vi "Filter ConfigurationView.vi"(9 "Stop Event":refnum<user-event>, 10 "Current Filter Settings":T1={"Level Filter"={"Warning"=FALSE, "Debug"=FALSE, "Info"=FALSE, "Error"=FALSE, "Critical"=FALSE}, "Source Filter"={"Source"="", "Exclude Match?"=TRUE, "Exact Match?"=TRUE}, "Keyword Filter"={"Keywords"=[], "Exclude Match?"=TRUE}}, 11 "ViewQueue":refnum<queue>) -> ()   [LabVIEW 2019, in "ConsoleView.lvlib" / "ConsoleView.lvclass"]
uses:
  <vilib>/gpm_packages/@cs/event-logger/Source/ConsoleView/View/ConsoleView.lvclass
  <vilib>/gpm_packages/@cs/event-logger/Source/Composed Log/Types/MessageCluster.ctl
  <vilib>/gpm_packages/@cs/event-logger/Source/ConsoleView/View/TypeDef/FilterConfig.ctl
  <vilib>/gpm_packages/@cs/event-logger/Source/Composed Log/Composed Log.lvlib
panel:
  in  "Cancel":bool
  in  "Apply Changes":bool
  in  "Exclude Keyword Matches?":bool caption="Exclude Matches?"
  in  "Exclude Source Matches?":bool caption="Exclude Matches?"
  in  "Exact Match?":bool
  in  "Keywords":string
  in  "Event Source":string
  in  "Critical":bool
  in  "Error":bool
  in  "Warning":bool
  in  "Info":bool
  in  "Debug":bool
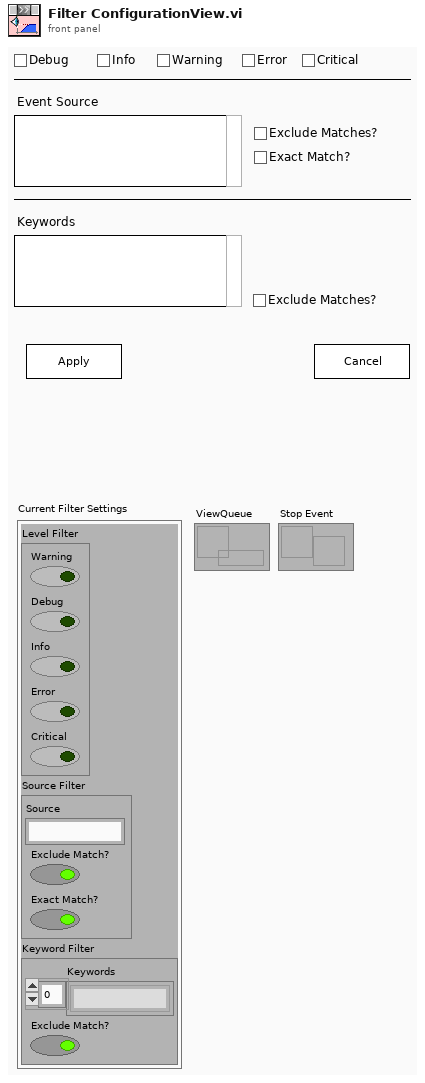
[diagram p1: front panel]
types:
  T1 = typedef "ConsoleView.lvlib/ConsoleView.lvclass/FilterConfig.ctl" = cluster{"Level Filter":cluster{"Warning":bool, "Debug":bool, "Info":bool, "Error":bool, "Critical":bool}, "Source Filter":cluster{"Source":string, "Exclude Match?":bool, "Exact Match?":bool}, "Keyword Filter":cluster{"Keywords":string[], "Exclude Match?":bool}}
  T2 = enum32{"Invalid", "Standard", "Closed", "Hidden", "Minimized", "Maximized"}
  T3 = typedef "Composed Log.lvlib/MessageCluster.ctl" = cluster{"Message":string, "Data":variant}
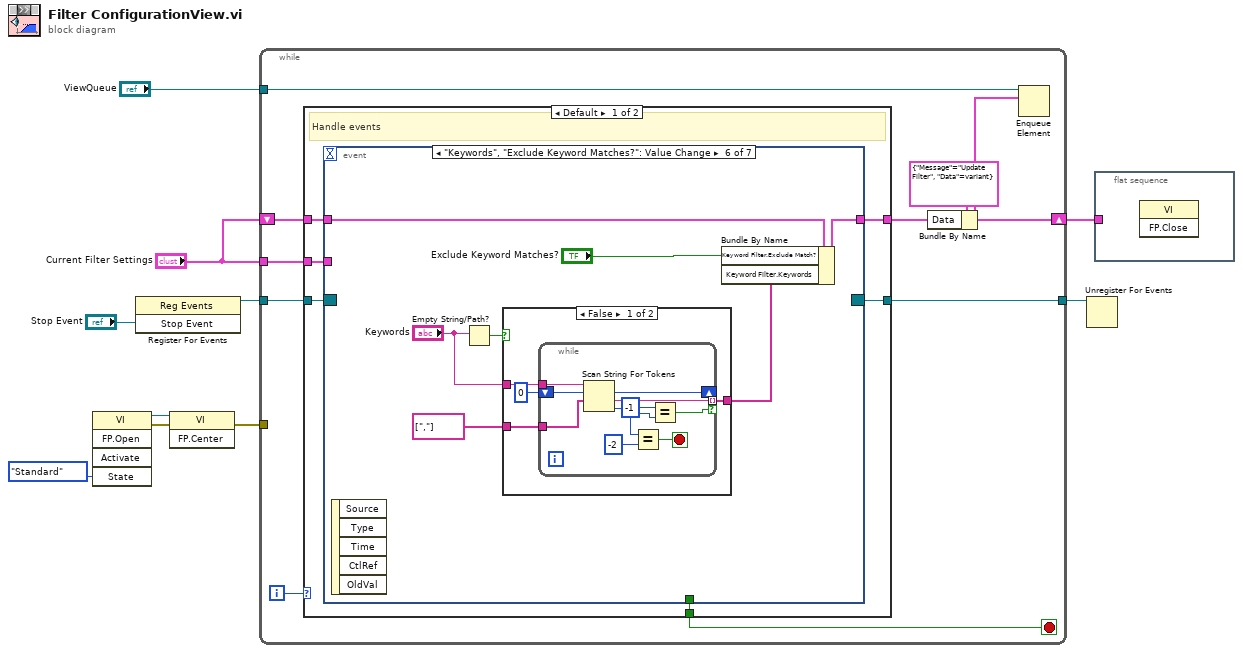
[diagram p0: block diagram]
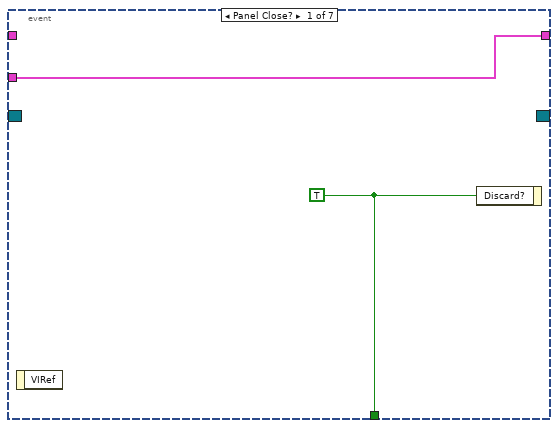
[diagram p2: hidden frame]
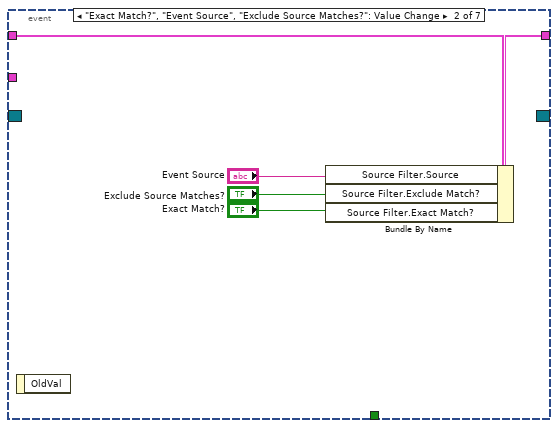
[diagram p3: hidden frame]
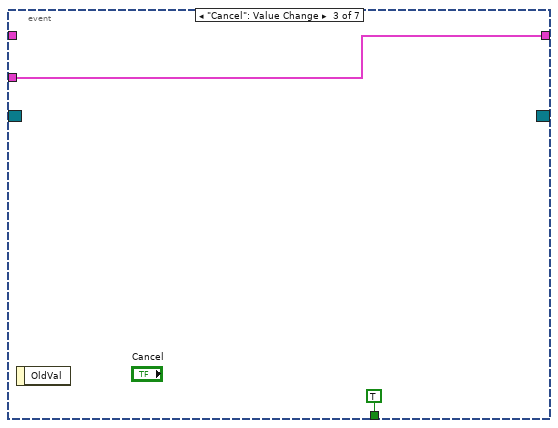
[diagram p4: hidden frame]
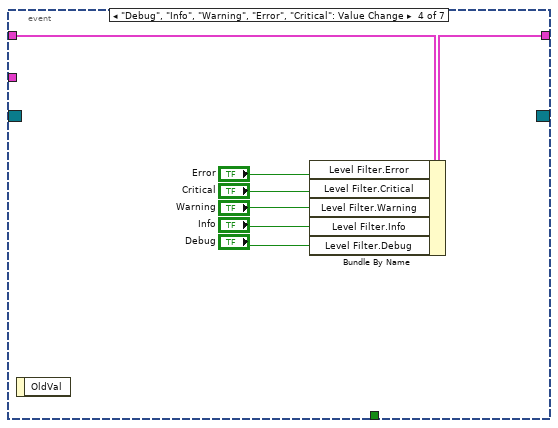
[diagram p5: hidden frame]
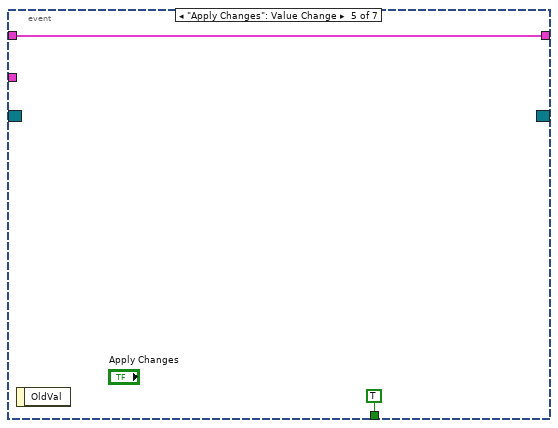
[diagram p6: hidden frame]
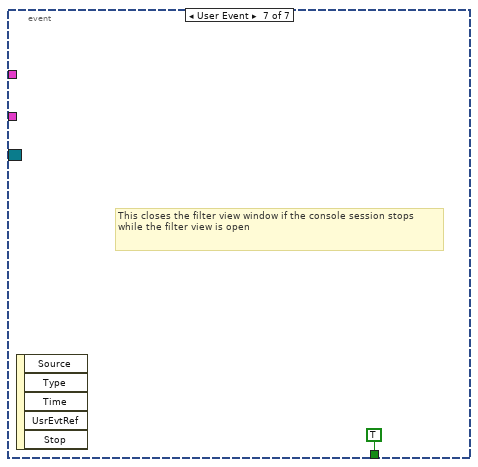
[diagram p8: hidden frame]
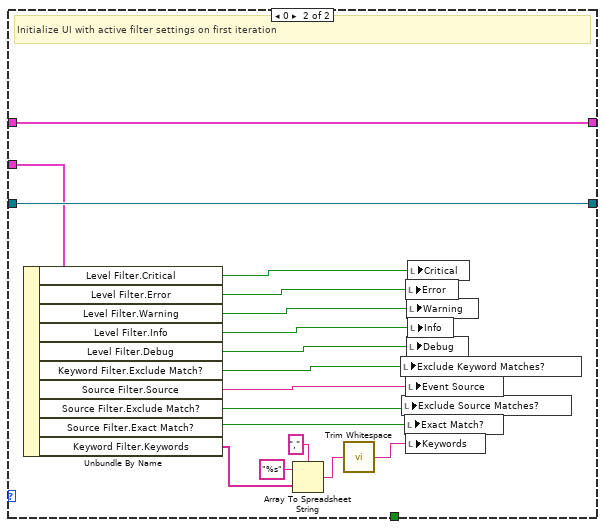
[diagram p9: hidden frame]
diagram:
  n1 = invoke class="VI" method="FP.Open"("State"=T2."Standard") -> (reference out=w7:refnum<vi>, error out=w6:errorcluster)  [unwired: 4 in, 3 out]
  n2 = register-events("Stop Event") -> (reference out=w2:refnum<event-registration>)  [unwired: 2 in, 1 out]
  n3 = invoke class="VI" method="FP.Center"(reference=w7, error in=w6) -> (error out=w5:errorcluster)  [unwired: 1 in, 2 out]
  n4 = while {
    shift-right: [w14] -> w4
    shift-left: "Current Filter Settings" -> [w19]
    tunnel: "Current Filter Settings" -> [w18]
    tunnel: "ViewQueue" -> [w17]
    tunnel: w5 -> [_]
    tunnel: w2 -> [w13]
    tunnel: [w12] -> w1
    i -> [w11]
    stop <- w20 stop-if-true
    n5 = case shown="Default" w11 {
      tunnel: [w26 _] -> w20
      tunnel: w19 -> [w25 w83]
      tunnel: w18 -> [w24 w81]
      tunnel: [w23 w83] -> w14
      tunnel: w13 -> [w22 w82]
      tunnel: [w21 w82] -> w12
      frame Default {
        # "Handle events"
        n6 = event shown="[5] \"Keywords\", \"Exclude Keyword Matches?\": Value Change" {
          selector: w22 -> [_ _ _ _ _ _ _]
          dyn-events: [_ _ _ _ _ _ _] -> w21
          timeout: _ -> [_ _ _ _ _ _ _]
          tunnel: [w28 _ TRUE ("Discard?") _ TRUE ("Discard?") _ TRUE ("Discard?")] -> w26
          tunnel: w25 -> [_ w33 _ w42 w44 w51 _]
          tunnel: [w27 w32 w35 w41 w44 w50 _] -> w23
          tunnel: w24 -> [w27 _ w35 _ _ _ _]
          event Panel Close? {
            w28 = TRUE ("Discard?")
            n7 = event-data() -> ()  [unwired: 1 in, 1 out]
            n8 = event-data("Discard?"=w28) -> ()  [unwired: 1 in, 1 out]
          }
          event "Exact Match?", "Event Source", "Exclude Source Matches?": Value Change {
            n9 = event-data() -> ()  [unwired: 1 in, 1 out]
            n10 = Bundle By Name(cluster=w33, "Source Filter.Source"="Event Source", "Source Filter.Exclude Match?"="Exclude Source Matches?", "Source Filter.Exact Match?"="Exact Match?") -> (w32:T1)
          }
          event "Cancel": Value Change {
            n11 = event-data() -> ()  [unwired: 1 in, 1 out]
          }
          event "Debug", "Info", "Warning", "Error", "Critical": Value Change {
            n12 = event-data() -> ()  [unwired: 1 in, 1 out]
            n13 = Bundle By Name(cluster=w42, "Level Filter.Error"="Error", "Level Filter.Critical"="Critical", "Level Filter.Warning"="Warning", "Level Filter.Info"="Info", "Level Filter.Debug"="Debug") -> (w41:T1)
          }
          event "Apply Changes": Value Change {
            n14 = event-data() -> ()  [unwired: 1 in, 1 out]
          }
          event "Keywords", "Exclude Keyword Matches?": Value Change {
            n15 = event-data() -> ()  [unwired: 1 in, 5 out]
            n16 = Empty String/Path?(string/path="Keywords") -> (empty?=w45:bool)
            n17 = case shown="False" w45 {
              tunnel: string[] [","] ("operators (none)") -> [w54 _]
              tunnel: "Keywords" -> [w53 _]
              tunnel: [w52 _] -> w46
              frame False {
                n18 = while {
                  tunnel: w53 -> [w65]
                  tunnel: [w64] -> w52 mode=indexing if=w57
                  shift-right: [w61] -> _
                  shift-left: 0 ("offset past token") -> [w60]
                  tunnel: w54 -> [w59]
                  stop <- w62 stop-if-true
                  n19 = Scan String For Tokens(7:w59, 8:w60, 9:w65) -> (0:w58:i32, 1:w64:string, 2:w61:i32)  [unwired: 3 in, 1 out]
                  n20 = Equal?(x=w58, y=-2) -> (x = y?=w62:bool)
                  n21 = Equal?(x=-1, y=w58) -> (x = y?=w57:bool)
                }
              }
              frame True {
              }
            }
            n22 = Bundle By Name(cluster=w51, "Keyword Filter.Exclude Match?"="Exclude Keyword Matches?", "Keyword Filter.Keywords"=w46) -> (w50:T1)
          }
          event User Event {
            # "This closes the filter view window if the console session stops while the filter view is open"
            n23 = event-data() -> ()  [unwired: 1 in, 5 out]
          }
        }
      }
      frame 0 {
        # "Initialize UI with active filter settings on first iteration"
        n24 = Unbundle By Name(w81) -> ("Level Filter.Critical"=w80:bool, "Level Filter.Error"=w79:bool, "Level Filter.Warning"=w78:bool, "Level Filter.Info"=w77:bool, "Level Filter.Debug"=w76:bool, "Keyword Filter.Exclude Match?"=w75:bool, "Source Filter.Source"=w71:string, "Source Filter.Exclude Match?"=w70:bool, "Source Filter.Exact Match?"=w69:bool, "Keyword Filter.Keywords"=w68:string[])
        n25 = Array To Spreadsheet String(delimiter (Tab)=",", array=w68, 3:"%s" ("format string")) -> (spreadsheet string=w72:string)
        n26 = call <vilib>:"Trim Whitespace.vi"("string"=w72) -> ("trimmed string"=w67:string)  [unwired: 1 in]
        n27 = local write "Exclude Keyword Matches?"(w75) -> ()
        n28 = local write "Exclude Source Matches?"(w70) -> ()
        n29 = local write "Exact Match?"(w69) -> ()
        n30 = local write "Error"(w79) -> ()
        n31 = local write "Event Source"(w71) -> ()
        n32 = local write "Keywords"(w67) -> ()
        n33 = local write "Warning"(w78) -> ()
        n34 = local write "Debug"(w76) -> ()
        n35 = local write "Critical"(w80) -> ()
        n36 = local write "Info"(w77) -> ()
      }
    }
    n37 = Bundle By Name(cluster=T3 {"Message"="Update Filter", "Data"=variant} ("element"), "Data"=w14) -> (w15:T3)
    n38 = Enqueue Element(queue=w17, element=w15) -> ()  [unwired: 2 in, 3 out]
  }
  n39 = Unregister For Events(event registration refnum=w1) -> ()  [unwired: 1 in, 1 out]
  n40 = flat-sequence {
    tunnel: w4 -> [_]
    frame #0 {
      n41 = invoke class="VI" method="FP.Close"() -> ()  [unwired: 3 in, 3 out]
    }
  }
